vi "Read Measurement (Initial Carrier Frequency).vi"(8 "error in (no error)":errorcluster, 9 "Maximum Time (20000 ms)":i32=20000, 11 "VISA resource name":refnum<visa-resource-name>) -> (0 "error out":errorcluster, 2 "Initial Carrier Frequency (Hz)":dbl, 3 "VISA resource name out":refnum<visa-resource-name>)   [LabVIEW 2014, in "Agilent ESA PSA Series.lvlib"]
doc: "Stops the present measurement and sets up the instrument for a spot frequency, initial carrier frequency measurement.\n\nAfter the data are valid, the result is returned for the specified measurement. These are the settings and units that conform to the measurement specific standard.\n\n- Stops the current measurement and does not reset the measurement to the factory defaults. \n\n- Initiates the measurement and puts valid data into the output buffer. If a measurement other than the current one is specified, the instrument will switch to that measurement before it initiates the measurement and returns results.\n\n- Waits until the measurement is complete before returning results.\n\n<B>Note:</B>\n\nThis VI is only valid for the Spot Frequency functionality of the Phase noise personality."
uses:
  Agilent ESA PSA Series.lvlib
  Fetch Measurement (Initial Carrier Frequency).vi
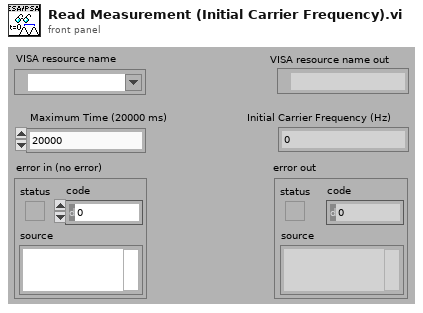
[diagram p1: front panel]
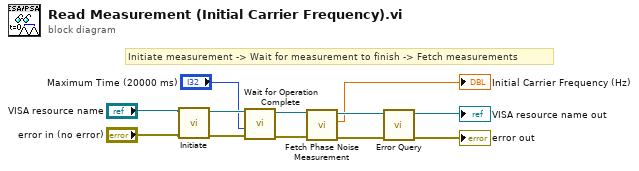
[diagram p0: block diagram]
diagram:
  # "Initiate measurement -> Wait for measurement to finish -> Fetch measurements"
  n1 = call "Initiate.vi"("error in (no error)"="error in (no error)", "VISA resource name"="VISA resource name") -> ("error out"=w9:errorcluster, "VISA resource name out"=w10:refnum<visa-resource-name>)  [unwired: 8 in]
  n2 = call "Wait for Operation Complete.vi"("error in (no error)"=w9, "Maximum Time (10000ms)"="Maximum Time (20000 ms)", "VISA resource name"=w10) -> ("error out"=w5:errorcluster, "VISA resource name out"=w6:refnum<visa-resource-name>)  [unwired: 7 in]
  n3 = call-poly "Fetch Phase Noise Measurement.vi"("error in (no error)"=w5, "VISA resource name"=w6) -> ("error out"=w3:errorcluster, "Initial Carrier Frequency (Hz)"=→"Initial Carrier Frequency (Hz)":dbl, "VISA resource name out"=w4:refnum<visa-resource-name>)  [unwired: 7 in]
  n4 = call "Error Query.vi"("error in (no error)"=w3, "VISA resource name"=w4) -> ("error out"=→"error out":errorcluster, "VISA resource name out"=→"VISA resource name out":refnum<visa-resource-name>)  [unwired: 6 in, 2 out]
